vi "niScope Read WDT.vi"(5 "timestamp Type":T1=1 caption="timestamp type" items=["relative", "absolute"], 7 "timeout":dbl=5.0 format="%.2f", 8 "error in":errorcluster, 9 "numSamples":i32=-1, 10 "channels":string="0", 11 "instrument handle":refnum<k15>) -> (0 "error out":errorcluster, 1 "wfm":waveform(dbl), 2 "wfm info":T2 {"reserved2" format="%.2f"; "reserved1" format="%.2f"; "offset" format="%^.3e"; "gain" format="%^.3e"; "xIncrement" format="%^.3e"; "relativeInitialX" format="%^.3e"; "absoluteInitialX" format="%^.3e"}, 3 "instrument handle out":refnum<k15>)   [LabVIEW 2011]
doc: "Returns the waveform the digitizer acquires for the specified channel. The VI initiates an acquisition that returns a scaled voltage waveform in a waveform data type that includes timing information."
uses:
  <instrlib>/niScope/Controls/niScope timestamp type.ctl
  niScope_32.dll
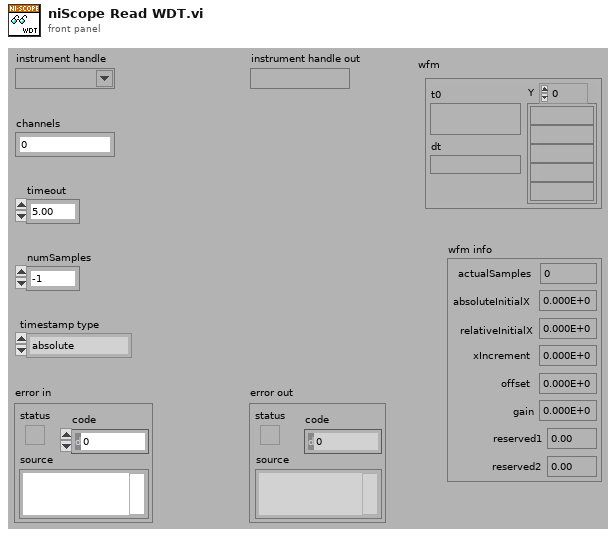
[diagram p1: front panel]
types:
  T1 = typedef "niScope timestamp type.ctl" = i32
  T2 = cluster{"actualSamples":i32, "absoluteInitialX":dbl, "relativeInitialX":dbl, "xIncrement":dbl, "offset":dbl, "gain":dbl, "reserved1":dbl, "reserved2":dbl}
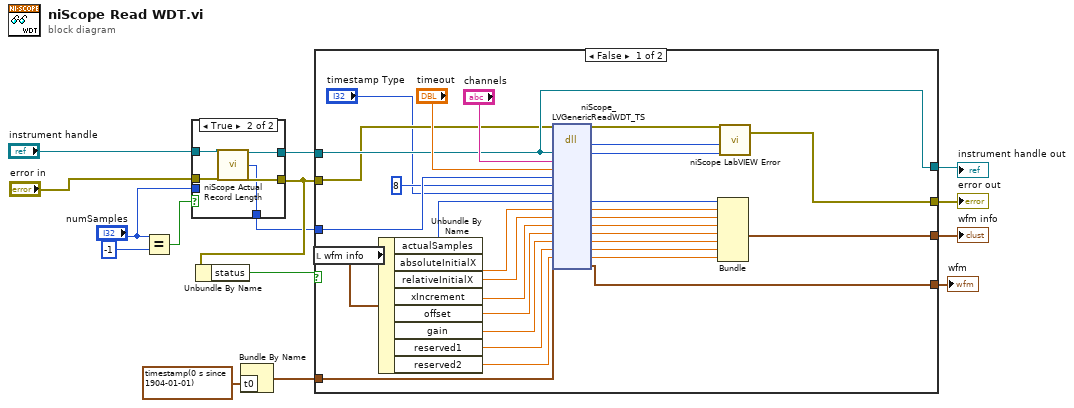
[diagram p0: block diagram]
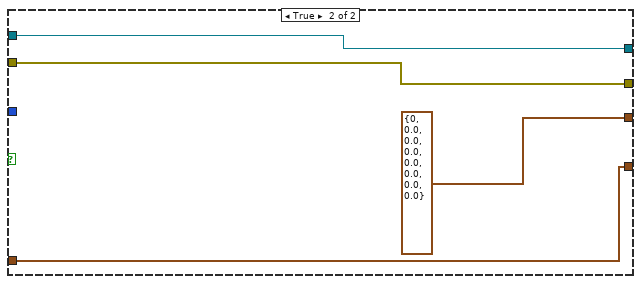
[diagram p3: hidden frame]
diagram:
  n1 = Equal?(x="numSamples", y=-1) -> (x = y?=w11:bool)
  n2 = case shown="True" w11 {
    tunnel: [w16 w23] -> w7
    tunnel: [w17 w22] -> w9
    tunnel: "numSamples" -> [w18 _]
    tunnel: [w18 w21] -> w6
    tunnel: "instrument handle" -> [w17 w20]
    tunnel: "error in" -> [w16 w19]
    frame False {
    }
    frame True {
      n3 = call <instrlib>:"niScope Actual Record Length.vi"("instrument handle"=w20, "error in"=w19) -> ("instrument handle out"=w22:refnum<k15>, "actual record length"=w21:i32, "error out"=w23:errorcluster)  [unwired: 11 in]
    }
  }
  n4 = Unbundle By Name(w7) -> ("status"=w13:bool)
  n5 = Bundle By Name("t0"=timestamp(0 s since 1904-01-01)) -> (w1:waveform(dbl))  [unwired: 1 in]
  n6 = case shown="False" w13 {
    tunnel: [w44 w57] -> w15
    tunnel: w9 -> [w47 w56]
    tunnel: w7 -> [w43 w57]
    tunnel: [w47 w56] -> w14
    tunnel: w6 -> [w51 _]
    tunnel: [w48 T2 {"actualSamples"=0, "absoluteInitialX"=0.0, "relativeInitialX"=0.0, "xIncrement"=0.0, "offset"=0.0, "gain"=0.0, "reserved1"=0.0, "reserved2"=0.0}] -> w8
    tunnel: [w34 w54] -> w3
    tunnel: w1 -> [w24 w54]
    frame False {
      n7 = local read "wfm info"() -> (w49:T2)
      n8 = Unbundle By Name(w49) -> ("actualSamples"=w35:i32, "absoluteInitialX"=w36:dbl, "relativeInitialX"=w37:dbl, "xIncrement"=w38:dbl, "offset"=w39:dbl, "gain"=w40:dbl, "reserved1"=w41:dbl, "reserved2"=w42:dbl)
      n9 = dll-call lib="niScope_*.*" fn="niScope_LVGenericReadWDT_TS"("instrument handle"=w47, "channel"="channels", "timeout"="timeout", "numSamples"=w51, "dataType"=8, "timestampType"="timestamp Type", "actualSamples"=w35, "absoluteInitialX"=w36, "relativeInitialX"=w37, "xIncrement"=w38, "offset"=w39, "gain"=w40, "reserved1"=w41, "reserved2"=w42, "wfm"=w24) -> ("status"=w46:i32, "instrument handle"=w45:u32, "actualSamples"=w26:i32, "absoluteInitialX"=w27:dbl, "relativeInitialX"=w28:dbl, "xIncrement"=w29:dbl, "offset"=w30:dbl, "gain"=w31:dbl, "reserved1"=w32:dbl, "reserved2"=w33:dbl, "wfm"=w34:waveform(dbl))  [unwired: 8 in, 2 out]
      n10 = Bundle("actualSamples"=w26, "absoluteInitialX"=w27, "relativeInitialX"=w28, "xIncrement"=w29, "offset"=w30, "gain"=w31, "reserved1"=w32, "reserved2"=w33) -> (w48:T2)  [unwired: 1 in]
      n11 = call <instrlib>:"niScope LabVIEW Error.vi"("instrument handle"=w45, "niScope error code (0)"=w46, "error in (no error)"=w43) -> ("error out"=w44:errorcluster)  [unwired: 2 in]
    }
    frame True {
    }
  }
  "instrument handle out" <- w14
  "error out" <- w15
  "wfm info" <- w8
  "wfm" <- w3
